vi "FITS_WriteImageU16.vi"(6 "Array":u16[](array[numeric])=[0, 0, 0, 0, 0, 0, 0, 0, 0, 0, 0, 0, 0, 0, 0, 0, 0, 0, 0, 0, 0, 0, 0, 0, 0, 0, 0, 0, 0, 0, 0, 0, 0, 0, 0, 0, 0, 0, 0, 0, 0, 0, 0, 0, 0, 0, 0, 0, 0, 0, 0, 0, 0, 0, 0, 1, 0, 0, 0, 0], 8 "error in":errorcluster, 9 "nelem":i32, 10 "firstel":i32, 11 "ref in":u64) -> (0 "error out":errorcluster, 2 "result":i32, 3 "ref out":u64)   [LabVIEW 2016]
uses:
  usr/local/lib/libfits.so
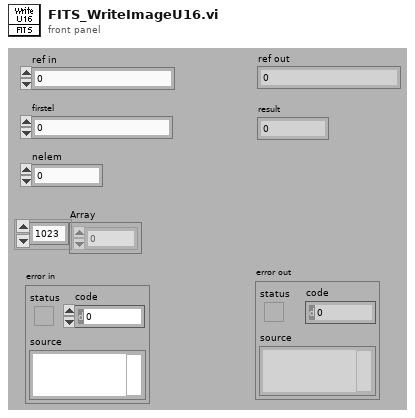
[diagram p1: front panel]
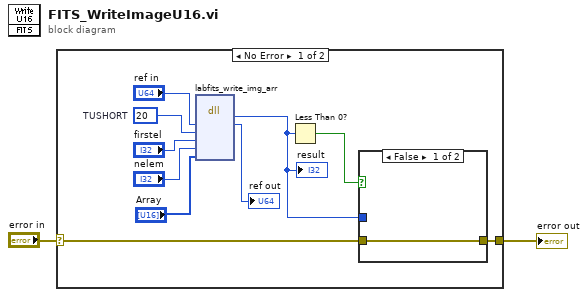
[diagram p0: block diagram]
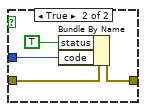
[diagram p2: hidden frame]
diagram:
  n1 = case shown="No Error" "error in" {
    selector: "error in" -> [w11 w18]
    tunnel: [w10 w18] -> w1
    frame No Error {
      w5 = 20  # TUSHORT
      n2 = dll-call lib="usr/local/lib/libfits.so" fn="labfits_write_img_arr"("ref"="ref in", "datatype"=w5, "firstel"="firstel", "nelem"="nelem", "data_array"="Array") -> ("return type"=w8:i32, "ref"=→"ref out":u64)  [unwired: 7 in, 2 out]
      "result" <- w8
      n3 = Less Than 0?(x=w8) -> (x < 0?=w12:bool)
      n4 = case shown="False" w12 {
        tunnel: w11 -> [w13 w15]
        tunnel: [w13 w14] -> w10
        tunnel: w8 -> [_ w16]
        frame False {
        }
        frame True {
          n5 = Bundle By Name(cluster=w15, "status"=TRUE, "code"=w16) -> (w14:errorcluster)
        }
      }
    }
    frame Error {
    }
  }
  "error out" <- w1
